vi "DAQmx Start Trigger (Analog Window).vi"(0 "task/channels in":refnum<k21>, 1 "when":i32(ring)=10163 items=["Entering Window"=10163, "Leaving Window"=10208], 5 "source":string, 7 "window top":dbl=0.5 format="%0.2f", 9 "window bottom":dbl format="%0.2f", 11 "error in":errorcluster) -> (4 "task out":refnum<k21>, 15 "error out":errorcluster)   [LabVIEW 2011]
doc: "Configures the task to start acquiring or generating samples when an analog signal enters or leaves a range you specify."
uses:
  C:/Program Files/National Instruments/LabVIEW 2011/resource/objmgr/daqmx.rc
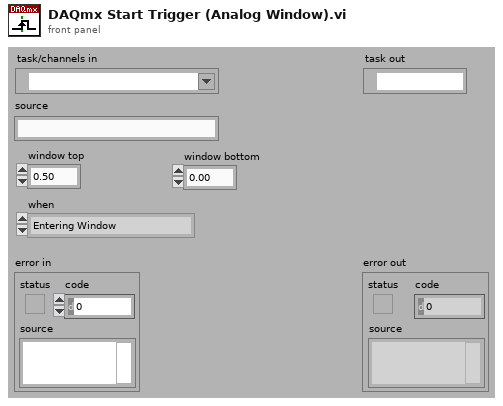
[diagram p1: front panel]
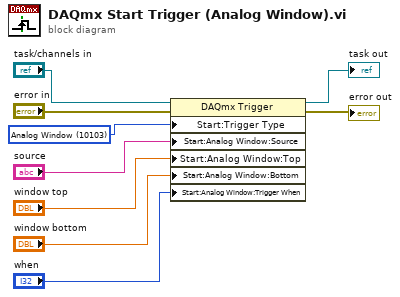
[diagram p0: block diagram]
diagram:
  w6 = 10103 items=["Analog Edge"=10099, "Digital Edge"=10150, "Analog Window"=10103, "None"=10230] ("Start:Trigger Type")
  n1 = property class="DAQmx Trigger"(reference="task/channels in", error in="error in", "Start:Trigger Type"=w6, "Start:Analog Window:Source"="source", "Start:Analog Window:Top"="window top", "Start:Analog Window:Bottom"="window bottom", "Start:Analog Window:Trigger When"="when") -> (reference out=→"task out":refnum<k21>, error out=→"error out":errorcluster)
